vi "Parse-ZIP-DOCX (SubVI).vi"(10 "Is ZIP":bool, 11 "Unknown File":path) -> (2 "Files Found":i32, 3 "ZIP Data":string[](array[string]))   [LabVIEW 2020]
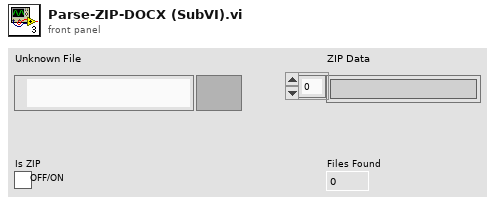
[diagram p1: front panel]
types:
  T1 = enum16{"open", "replace", "create", "open or create", "replace or create", "replace or create with confirmation"}
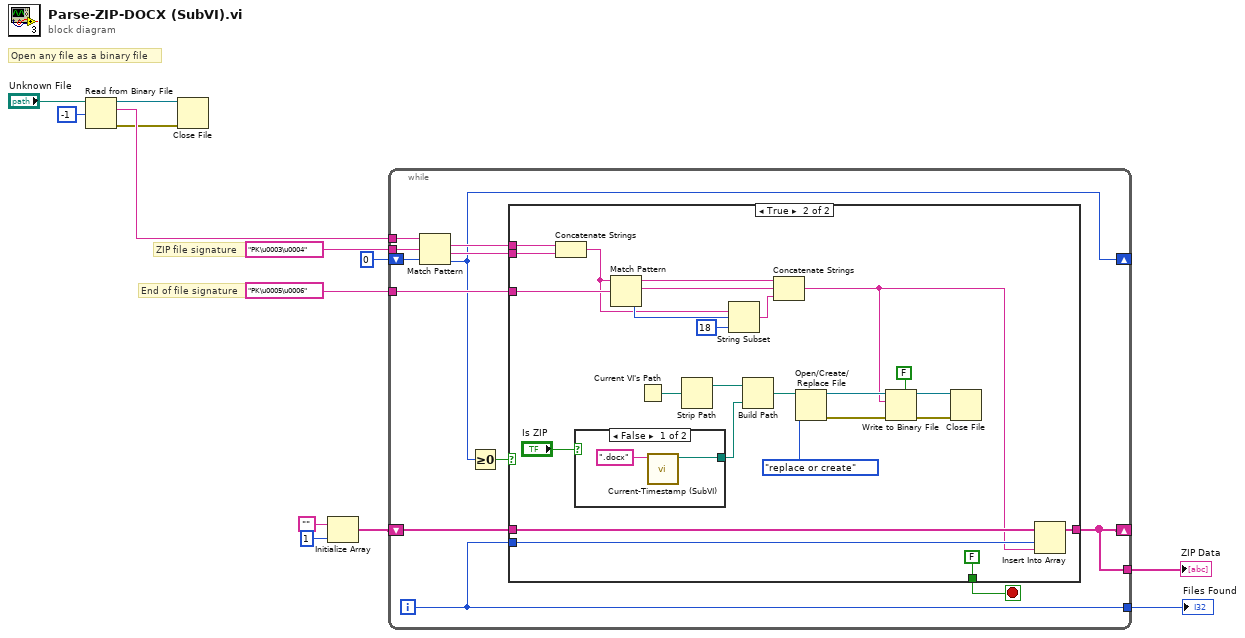
[diagram p0: block diagram]
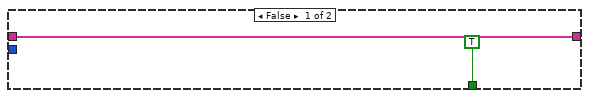
[diagram p2: hidden frame]
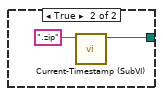
[diagram p3: hidden frame]
diagram:
  # "End of file signature"
  # "ZIP file signature"
  # "Open any file as a binary file"
  n1 = Read from Binary File(10:-1 ("count (1)"), 11:"Unknown File") -> (0:w4:errorcluster, 2:w6:string, 3:w3:refnum<file>)  [unwired: 4 in, 1 out]
  n2 = Close File(refnum=w3, error in=w4) -> ()  [unwired: 2 out]
  n3 = Initialize Array("", 1 ("dimension size")) -> (w9:string[])
  n4 = while {
    tunnel: "PK\u0003\u0004" -> [w21]
    tunnel: "PK\u0005\u0006" -> [w25]
    tunnel: w6 -> [w22]
    shift-right: [w17] -> _
    shift-left: 0 -> [w18]
    shift-right: [w15] -> _
    shift-left: w9 -> [w16]
    tunnel: [w15] -> w10
    tunnel: [w14] -> w11
    i -> [w14]
    stop <- w23 stop-if-true
    n5 = Match Pattern(string=w22, regular expression=w21, offset (0)=w18) -> (match substring=w20:string, after substring=w19:string, offset past match=w17:i32)  [unwired: 1 out]
    n6 = Greater Or Equal To 0?(x=w17) -> (x >= 0?=w24:bool)
    n7 = case shown="True" w24 {
      tunnel: w25 -> [_ w43]
      tunnel: [TRUE FALSE] -> w23
      tunnel: w20 -> [_ w41]
      tunnel: w19 -> [_ w40]
      tunnel: w16 -> [w26 w39]
      tunnel: w14 -> [_ w38]
      tunnel: [w26 w37] -> w15
      frame False {
      }
      frame True {
        n8 = Concatenate Strings(w41, w40) -> (w30:string)
        n9 = case shown="False" "Is ZIP" {
          tunnel: [w53 w55] -> w35
          frame False {
            n10 = call "Current-Timestamp (SubVI).vi"("Extension"=".docx" ("string")) -> ("Path"=w53:path)  [unwired: 10 in]
          }
          frame True {
            n11 = call "Current-Timestamp (SubVI).vi"("Extension"=".zip" ("string")) -> ("Path"=w55:path)  [unwired: 10 in]
          }
        }
        n12 = Match Pattern(string=w30, regular expression=w43) -> (before substring=w29:string, match substring=w28:string, offset past match=w31:i32)  [unwired: 1 in, 1 out]
        n13 = Current VI's Path() -> (path=w48:path)
        n14 = Strip Path(path=w48) -> (stripped path=w47:path)  [unwired: 1 out]
        n15 = String Subset(string=w30, offset (0)=w31, length (rest)=18 ("length (rest)")) -> (substring=w34:string)
        n16 = Build Path(base path=w47, name or relative path=w35) -> (appended path=w46:path)
        n17 = Concatenate Strings(w29, w28, w34) -> (w32:string)
        n18 = Open/Create/Replace File(file path (use dialog)=w46, operation (0:open)=T1."replace or create") -> (refnum out=w45:refnum<file>, error out=w51:errorcluster)  [unwired: 4 in, 1 out]
        n19 = Write to Binary File(file (use dialog)=w45, data=w32, error in=w51, 5:FALSE ("prepend array or string size? (T)")) -> (refnum out=w49:refnum<file>, error out=w50:errorcluster)  [unwired: 2 in, 1 out]
        n20 = Close File(refnum=w49, error in=w50) -> ()  [unwired: 2 out]
        n21 = Insert Into Array(array=w39, index=w38, new element=w32) -> (w37:string[])
      }
    }
  }
  "ZIP Data" <- w10
  "Files Found" <- w11
